vi "Read Math.vi"(8 "error in (no error)":errorcluster, 10 "Reset After Read (False)":bool, 11 "VISA resource name":refnum<visa-resource-name>) -> (0 "error out":errorcluster, 1 "Count":dbl, 2 "Average":dbl, 3 "VISA resource name out":refnum<visa-resource-name>, 5 "Minimum":dbl, 7 "Maximum":dbl)   [LabVIEW 2020, in "Agilent 34405.lvlib"]
doc: "Read Math returns the minimum, maximum, average, count from multiple measurements. This VI requires that Min/Max is set in Configure Math and should be called after multiple measurements have been taken."
uses:
  <instrlib>/Agilent 34405/Agilent 34405.lvlib
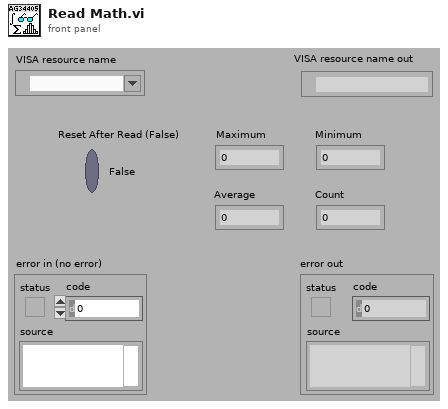
[diagram p1: front panel]
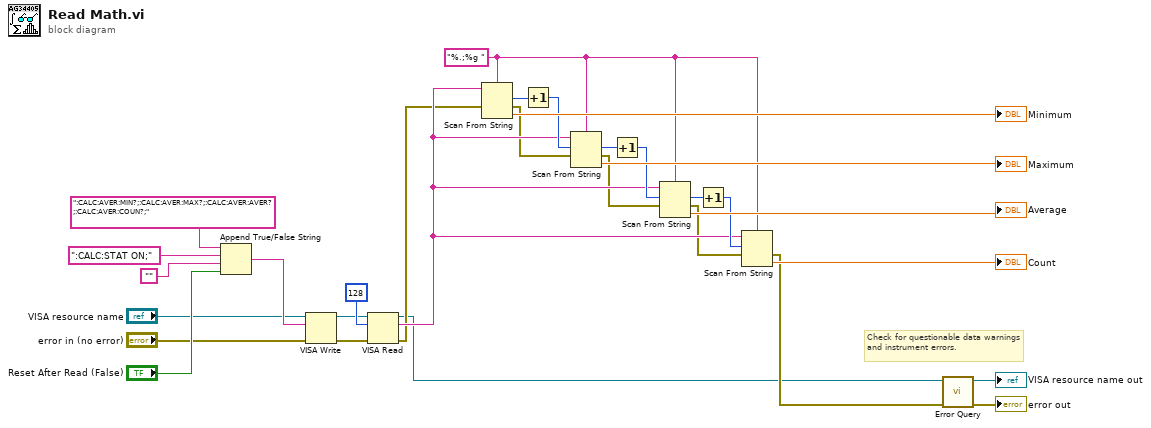
[diagram p0: block diagram]
diagram:
  w10 = "%.;%g " ("format string")
  # "Check for questionable data warnings and instrument errors."
  n1 = Append True/False String(1:"Reset After Read (False)", 2:"" ("Empty String Constant"), 3:":CALC:STAT ON;", 4:":CALC:AVER:MIN?;:CALC:AVER:MAX?;:CALC:AVER:AVER?;:CALC:AVER:COUN?;") -> (0:w20:string)
  n2 = VISA Write(VISA resource name="VISA resource name", write buffer=w20, error in (no error)="error in (no error)") -> (VISA resource name out=w17:refnum<visa-resource-name>, error out=w18:errorcluster)  [unwired: 1 out]
  n3 = VISA Read(VISA resource name=w17, byte count=u32 128, error in (no error)=w18) -> (VISA resource name out=w1:refnum<visa-resource-name>, read buffer=w9:string, error out=w8:errorcluster)  [unwired: 1 out]
  n4 = Scan From String(format string=w10, input string=w9, error in=w8) -> (offset past scan=w11:u32, error out=w7:errorcluster, output 1=→"Minimum":dbl)  [unwired: 1 in, 2 out]
  n5 = Increment(x=w11) -> (x+1=w12:u32)
  n6 = Scan From String(format string=w10, input string=w9, initial scan location=w12, error in=w7) -> (offset past scan=w13:u32, error out=w6:errorcluster, output 1=→"Maximum":dbl)  [unwired: 2 out]
  n7 = Increment(x=w13) -> (x+1=w14:u32)
  n8 = Scan From String(format string=w10, input string=w9, initial scan location=w14, error in=w6) -> (offset past scan=w15:u32, error out=w5:errorcluster, output 1=→"Average":dbl)  [unwired: 2 out]
  n9 = Increment(x=w15) -> (x+1=w16:u32)
  n10 = Scan From String(format string=w10, input string=w9, initial scan location=w16, error in=w5) -> (error out=w2:errorcluster, output 1=→"Count":dbl)  [unwired: 1 in, 2 out]
  n11 = call <instrlib>:"Error Query.vi"("error in (no error)"=w2, "VISA resource name"=w1) -> ("error out"=→"error out":errorcluster, "VISA resource name out"=→"VISA resource name out":refnum<visa-resource-name>)  [unwired: 8 out]
